vi "Parse Xml Node Recursively from File.vi"(8 "error in":errorcluster, 9 "Parents":string[](array[string]), 10 "Path to XML document":path, 11 "Item Data":refnum<class "Item.lvclass">[](array[class])) -> (0 "error out":errorcluster, 3 "Item Data out":refnum<class "Item.lvclass">[](array[class]))   [LabVIEW 2020, in "VI Properties Editor.lvlib"]
doc: "This VI is meant to be used to parse xml files like classes and lvlib that are nested members of a lvlib or one of it's members."
uses:
  VI Properties Editor.lvlib
  <vilib>/xml/NI_XML.lvlib
  <vilib>/xml/Load XML String.vi
  <vilib>/xml/Close Reference(Node).vi
  Classes/Item/Item.lvclass
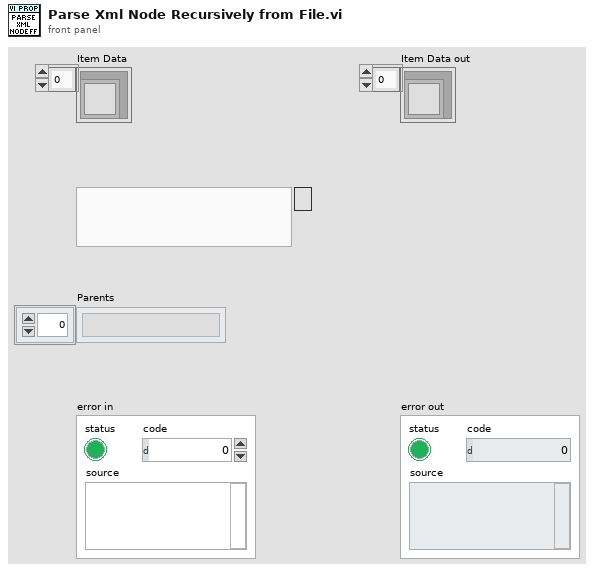
[diagram p1: front panel]
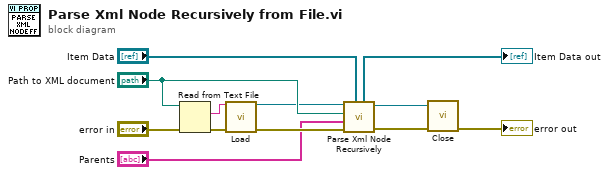
[diagram p0: block diagram]
diagram:
  n1 = Read from Text File(file (use dialog)="Path to XML document", error in="error in") -> (text=w10:string, error out=w11:errorcluster)  [unwired: 2 in, 2 out]
  n2 = call-poly <vilib>:"Load.vi"("XML string"=w10, "error in (no error)"=w11) -> ("DOM document out"=w7:refnum<k20>, "error out"=w8:errorcluster)  [unwired: 11 in, 1 out]
  n3 = call "Parse Xml Node Recursively.vi"("Item Data"="Item Data", "error in"=w8, "Parents"="Parents", "XML File Path"="Path to XML document", "Node in"=w7) -> ("error out"=w6:errorcluster, "Node out"=w3:refnum<k20>, "Item Data out"=→"Item Data out":refnum<class "Item.lvclass">[])  [unwired: 4 in]
  n4 = call-poly <vilib>:"Close.vi"("error in (no error)"=w6, "node"=w3) -> ("error out"=→"error out":errorcluster)  [unwired: 7 in]
